vi "Get Property Access.vi"(0 "SLSC Remote in":refnum<class "SLSC Remote.lvclass">, 5 "property":refnum<k21>, 11 "error in (no error)":errorcluster) -> (4 "SLSC Remote out":refnum<class "SLSC Remote.lvclass">, 6 "property out":refnum<k21>, 10 "Prop.Access":i32(ring) items=["None", "Read Only", "Write Only", "Read/Write"], 15 "error out":errorcluster)   [LabVIEW 2016, in "SLSC Interfaces.lvlib" / "SLSC Remote.lvclass"]
uses:
  SLSC Remote.lvclass
  C:/Users/tblair/Documents/SLSC-Interface/Source/SLSC Interface Class/SLSC Interface.lvclass
  <vilib>/rajsite/i3-json/JSON Generation/Create Value Files/Create Value - Object.vi
  <vilib>/rajsite/i3-json/JSON Generation/Add Object Parameter Files/Add Object Parameter - String.vi
  <vilib>/NI/NI JSONRPC Server Framework/Classes/Server/Format Client Request (Auto-Increment).vi
  <vilib>/httpClient/POSTBuffer.vi
  <vilib>/rajsite/i3-json/JSON Parsing/Get Object Parameter Files/Get Object Parameter - String.vi
  <vilib>/NI/NI JSONRPC Server Framework/Classes/Server/JSONRPC Server.lvclass
  <vilib>/rajsite/i3-json/i3-json.lvlib
  <vilib>/httpClient/LabVIEWHTTPClient.lvlib
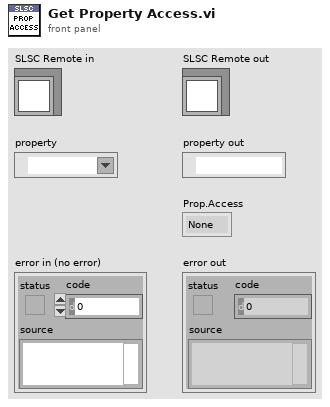
[diagram p1: front panel]
types:
  T1 = typedef "LabVIEWHTTPClient.lvlib/ClientHandle.ctl" = refnum<k1>
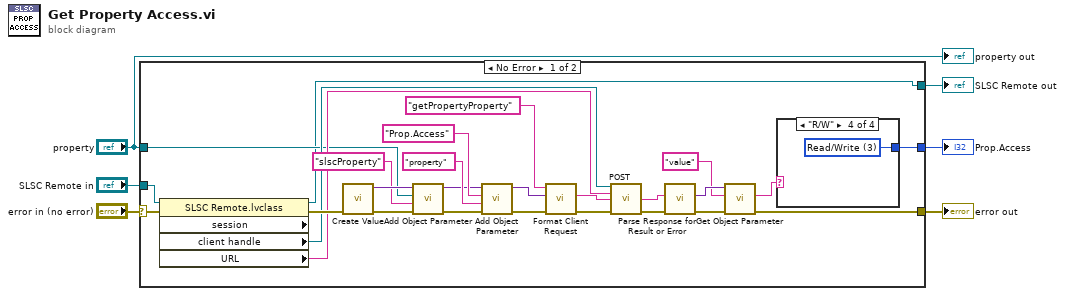
[diagram p0: block diagram]
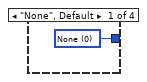
[diagram p2: hidden frame]
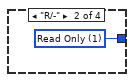
[diagram p3: hidden frame]
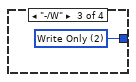
[diagram p4: hidden frame]
diagram:
  n1 = case shown="No Error" "error in (no error)" {
    selector: "error in (no error)" -> [w31 w39]
    tunnel: "SLSC Remote in" -> [w32 w38]
    tunnel: [w19 w39] -> w3
    tunnel: "property" -> [w13 _]
    tunnel: [w8 _] -> w4
    tunnel: [w7 w38] -> w1
    frame No Error {
      n2 = property class="SLSC Remote.lvclass" props=["session", "client handle", "URL"](reference=w32, error in=w31) -> (reference out=w7:refnum<class "SLSC Remote.lvclass">, error out=w30:errorcluster, "client handle"=w26:T1, "URL"=w25:string)  [unwired: 1 out]
      n3 = call-poly <vilib>:"Create Value.vi"("error in (no error)"=w30) -> ("error out"=w29:errorcluster, "JSON Tree"=w33:variant)  [unwired: 9 in]
      n4 = call-poly <vilib>:"Add Object Parameter.vi"("error in (no error)"=w29, "Name"="slscProperty", "String"=w13, "JSON Tree in (JSON Object)"=w33) -> ("error out"=w10:errorcluster, "JSON Tree out (JSON Object)"=w11:variant)  [unwired: 6 in]
      n5 = call-poly <vilib>:"Add Object Parameter.vi"("error in (no error)"=w10, "Name"="property", "String"="Prop.Access", "JSON Tree in (JSON Object)"=w11) -> ("error out"=w16:errorcluster, "JSON Tree out (JSON Object)"=w17:variant)  [unwired: 6 in]
      n6 = call-poly <vilib>:"Format Client Request.vi"("error in (no error)"=w16, "params"=w17, "method"="getPropertyProperty") -> ("error out"=w24:errorcluster, "Request String"=w27:string)  [unwired: 7 in]
      n7 = call-poly <vilib>:"POST.vi"("client handle"=w26, "url"=w25, "buffer"=w27, "error in (no error)"=w24) -> ("body"=w23:string, "error out"=w22:errorcluster)  [unwired: 8 in, 2 out]
      n8 = call <vilib>:"Parse Response for Result or Error.vi"("error in"=w22, "Response String In"=w23) -> ("error out"=w20:errorcluster, "Result or Error Data"=w21:variant)  [unwired: 7 in, 1 out]
      n9 = call-poly <vilib>:"Get Object Parameter.vi"("error in (no error)"=w20, "Parameter Name"="value", "JSON Tree In (JSON Object)"=w21) -> ("error out"=w19:errorcluster, "String Value"=w9:string)  [unwired: 5 in, 2 out]
      n10 = case shown="\"R/W\"" w9 {
        tunnel: [w34 w35 w36 w37] -> w8
        frame "None", Default {
          w34 = 0 items=["None", "Read Only", "Write Only", "Read/Write"] ("Prop.Access")
        }
        frame "R/-" {
          w35 = 1 items=["None", "Read Only", "Write Only", "Read/Write"] ("Prop.Access")
        }
        frame "-/W" {
          w36 = 2 items=["None", "Read Only", "Write Only", "Read/Write"] ("Prop.Access")
        }
        frame "R/W" {
          w37 = 3 items=["None", "Read Only", "Write Only", "Read/Write"] ("Prop.Access")
        }
      }
    }
    frame Error {
    }
  }
  "error out" <- w3
  "SLSC Remote out" <- w1
  "Prop.Access" <- w4
  "property out" <- "property"
